vi "Set Operational Mode.vi"(7 "Box ID":u8, 8 "error in (no error)":errorcluster, 9 "Precision Mode":bool, 10 "PID Disable":bool, 11 "BS120x in":refnum<class "BS120x.lvclass">) -> (0 "error out":errorcluster, 3 "BS120x out":refnum<class "BS120x.lvclass">)   [LabVIEW 2021, in "BS120x Driver.lvlib" / "BS120x.lvclass"]
uses:
  BS120x.lvclass
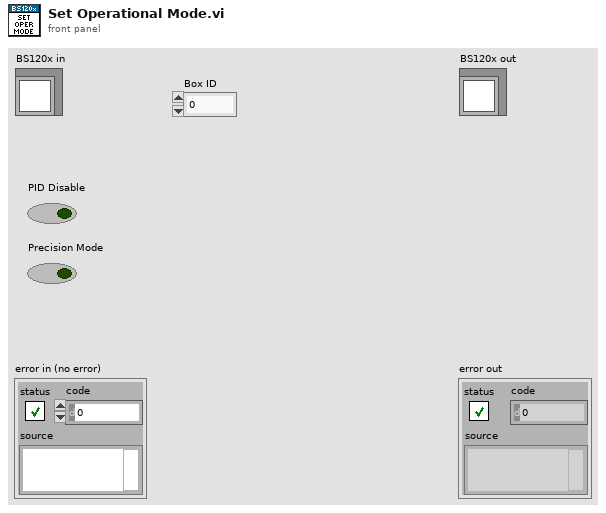
[diagram p1: front panel]
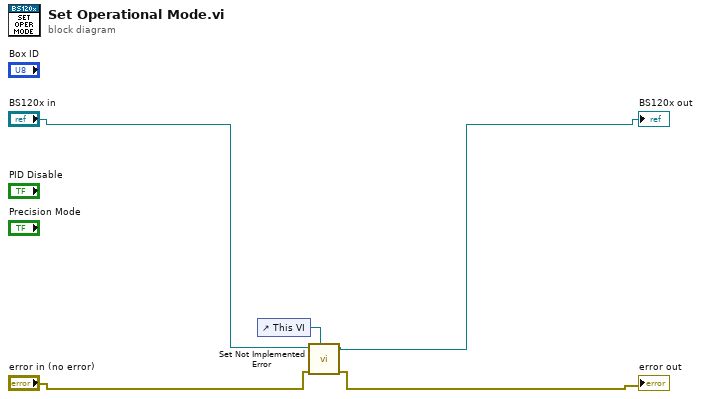
[diagram p0: block diagram]
diagram:
  n1 = control-ref of="This VI"() -> (w5:refnum<vi>)
  n2 = call "Set Not Implemented Error.vi"("VI Reference"=w5, "error in (no error)"="error in (no error)", "BS120x in"="BS120x in") -> ("error out"=→"error out":errorcluster, "BS120x out"=→"BS120x out":refnum<class "BS120x.lvclass">)  [unwired: 7 in]
